vi "新建通讯互斥锁.vi"(8 "error in (no error)":errorcluster) -> (0 "error out":errorcluster)   [LabVIEW 2016, in "斯坦道总磷总氮.lvlib"]
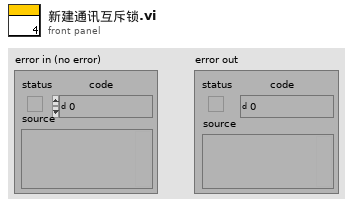
[diagram p1: front panel]
types:
  T1 = typedef "Semaphore RefNum" = refnum<k1>
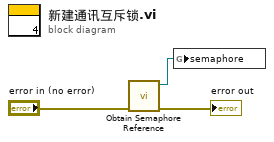
[diagram p0: block diagram]
diagram:
  n1 = call <vilib>:"Obtain Semaphore Reference.vi"("error in (no error)"="error in (no error)") -> ("error out"=→"error out":errorcluster, "semaphore"=w1:T1)  [unwired: 4 in, 1 out]
  n2 = global write "VAR总磷总氮全局变量.vi" "semaphore"(w1) -> ()
